vi "powermeter-init.vi"(0 "VISA in":refnum<visa-resource-name>) -> (1 "Powermeter initialization ok?":bool, 2 "VISA out":refnum<visa-resource-name>, 3 "error out":errorcluster)   [LabVIEW 2017]
doc: "This VI scans for connected devices, that can be selected in a dialog box. Next steps\n- setting timeout\n- performing identification query\n- configuring the operation register to '512'; flag gets to HI when a new measurement value is ready to fetch\n- clear operation register"
panel:
  out "status":bool
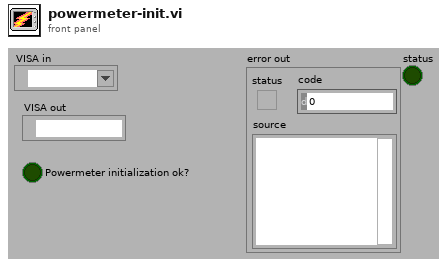
[diagram p1: front panel]
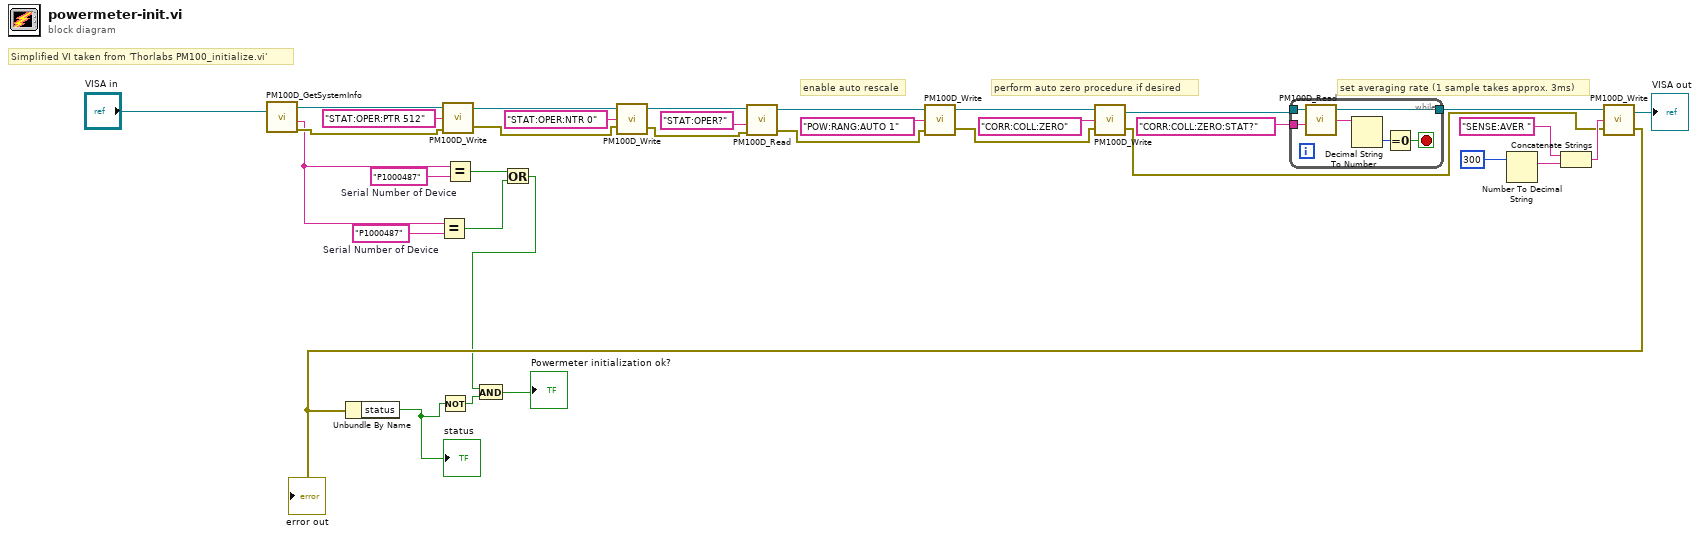
[diagram p0: block diagram]
diagram:
  w3 = "P1000487"  # Serial Number of Device
  w30 = "P1000487"  # Serial Number of Device
  # "set averaging rate (1 sample takes approx. 3ms)"
  # "enable auto rescale"
  # "perform auto zero procedure if desired"
  # "Simplified VI taken from 'Thorlabs PM100_initialize.vi'"
  n1 = call "PM100D_GetSystemInfo.vi"("VISA in"="VISA in") -> ("VISA out"=w34:refnum<visa-resource-name>, "SN"=w2:string, "error out"=w8:errorcluster)  [unwired: 1 in, 1 out]
  n2 = Equal?(x=w2, y=w3) -> (x = y?=w1:bool)
  n3 = call "PM100D_Write.vi"("error in (no error)"=w8, "Command"="STAT:OPER:PTR 512", "VISA in"=w34) -> ("error out"=w14:errorcluster, "VISA out"=w33:refnum<visa-resource-name>)
  n4 = Equal?(x=w2, y=w30) -> (x = y?=w5:bool)
  n5 = Or(x=w5, y=w1) -> (x .or. y?=w4:bool)
  n6 = call "PM100D_Write.vi"("error in (no error)"=w14, "Command"="STAT:OPER:NTR 0", "VISA in"=w33) -> ("error out"=w12:errorcluster, "VISA out"=w31:refnum<visa-resource-name>)
  n7 = call "PM100D_Read.vi"("error in (no error)"=w12, "Command"="STAT:OPER?", "VISA in"=w31) -> ("error out"=w11:errorcluster, "VISA out"=w28:refnum<visa-resource-name>)  [unwired: 1 in, 1 out]
  n8 = call "PM100D_Write.vi"("error in (no error)"=w11, "Command"="POW:RANG:AUTO 1" ("string"), "VISA in"=w28) -> ("error out"=w10:errorcluster, "VISA out"=w26:refnum<visa-resource-name>)
  n9 = call "PM100D_Write.vi"("error in (no error)"=w10, "Command"="CORR:COLL:ZERO" ("string"), "VISA in"=w26) -> ("error out"=w9:errorcluster, "VISA out"=w25:refnum<visa-resource-name>)
  n10 = while {
    tunnel: "CORR:COLL:ZERO:STAT?" ("string") -> [w40]
    tunnel: w25 -> [w41]
    tunnel: [w39] -> w19
    stop <- w36 stop-if-true
    n11 = call "PM100D_Read.vi"("Command"=w40, "VISA in"=w41) -> ("ReadValue"=w38:string, "VISA out"=w39:refnum<visa-resource-name>)  [unwired: 2 in, 1 out]
    n12 = Decimal String To Number(string=w38) -> (number=w37:i32)  [unwired: 2 in, 1 out]
    n13 = Equal To 0?(x=w37) -> (x = 0?=w36:bool)
  }
  n14 = Number To Decimal String(number=300) -> (decimal integer string=w22:string)  [unwired: 1 in]
  n15 = Concatenate Strings("SENSE:AVER " ("string"), w22) -> (w21:string)
  n16 = call "PM100D_Write.vi"("error in (no error)"=w9, "Command"=w21, "VISA in"=w19) -> ("error out"=w7:errorcluster, "VISA out"=→"VISA out":refnum<visa-resource-name>)
  "error out" <- w7
  n17 = Unbundle By Name(w7) -> ("status"=w16:bool)
  "status" <- w16
  n18 = Not(x=w16) -> (.not. x?=w17:bool)
  n19 = And(x=w4, y=w17) -> (x .and. y?=→"Powermeter initialization ok?":bool)
